vi "Trace.vi"(8 "Error In":errorcluster, 11 "Text":string) -> (0 "Error Out":errorcluster)   [LabVIEW 2015, in "Logger.lvlib"]
doc: "Creates a logging statement from a message string with the TRACE level. The statement is created even if an error is passed to the Error In terminal. The logging level must be set to six (6) or higher for this statement to be received by listeners. A logging statement is a comma-separated values (CSV) line containing an ISO 8601 timestamp, the level name (\"TRACE\"), the name of the origin VI, and the message."
uses:
  Logger.lvlib
  Private/Action.ctl
  Controls/Message.ctl
  Controls/Tag.ctl
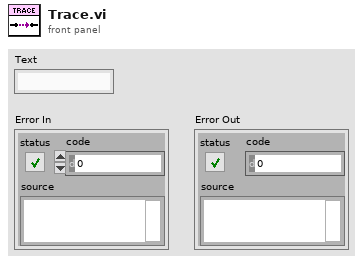
[diagram p1: front panel]
types:
  T1 = typedef "Logger.lvlib/Tag.ctl" = enum16{"Fatal", "Error", "Warn", "Info", "Debug", "Trace"}
  T2 = typedef "Logger.lvlib/Message.ctl" = cluster{"Time Stamp":timestamp, "Tag":T1, "Source":string, "Text":string}
  T3 = typedef "Logger.lvlib/Action.ctl" = enum16{"Initialize", "Register", "Log", "Unregister", "Set Level", "Shutdown"}
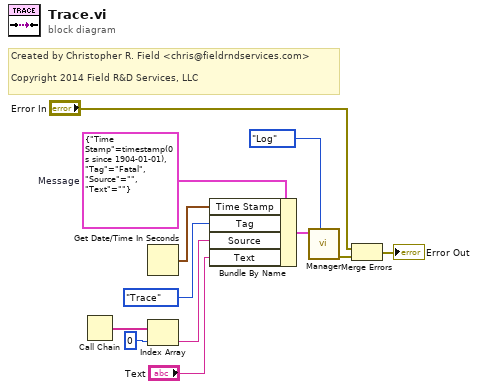
[diagram p0: block diagram]
diagram:
  w7 = T2 {"Time Stamp"=timestamp(0 s since 1904-01-01), "Tag"=enum."Fatal", "Source"="", "Text"=""}  # Message
  # "Created by Christopher R. Field <chris@fieldrndservices.com>\n\nCopyright 2014 Field R&D Services, LLC"
  n1 = Call Chain() -> (call chain=w9:string[])
  n2 = Get Date/Time In Seconds() -> (seconds since 1Jan1904=w6:timestamp)
  n3 = Index Array(array=w9, index=0) -> (element=w4:string)
  n4 = Bundle By Name(cluster=w7, "Time Stamp"=w6, "Tag"=Tag."Trace" ("Level"), "Source"=w4, "Text"="Text") -> (w3:T2)
  n5 = call "Manager.vi"("Action"=Action."Log", "Value In"=w3) -> ("Error Out"=w12:errorcluster)  [unwired: 9 in]
  n6 = Merge Errors("Error In", w12) -> (→"Error Out":errorcluster)
